vi "Drive Controller.vi"(8 "error in":errorcluster) -> ()   [LabVIEW 2015]
doc: "This VI executes continuously carrying out the current operation and responding to updates or new operation requests. It will often contain the timing or control code that is difficult to place directly in TeleOp. This VI generally opens all sensors and motors and isolates the rest of the robot code from knowing implementation details of how the operations are carried out."
uses:
  JoystickData.ctl
  Drive Setpoints.ctl
  Drive Operations.ctl
  Framework/Robot Global Data.vi
  Global Drive Variables.vi
  RobotDriveGlobal.vi
panel:
  out "Waveform Chart":cluster{"output":dbl, "Angle":dbl, "Yaw":dbl}(graph)
  out "Setpoints":T1(graph)
  out "Current\nCmd":string
  # "Tip: It may be helpful to observe inputs and sensor values.\nYou may also want to display tuning or debugging controls."
  # "Working PID Values:\nP:\nI:\nD:\nF:\nIZ:\nRR:"
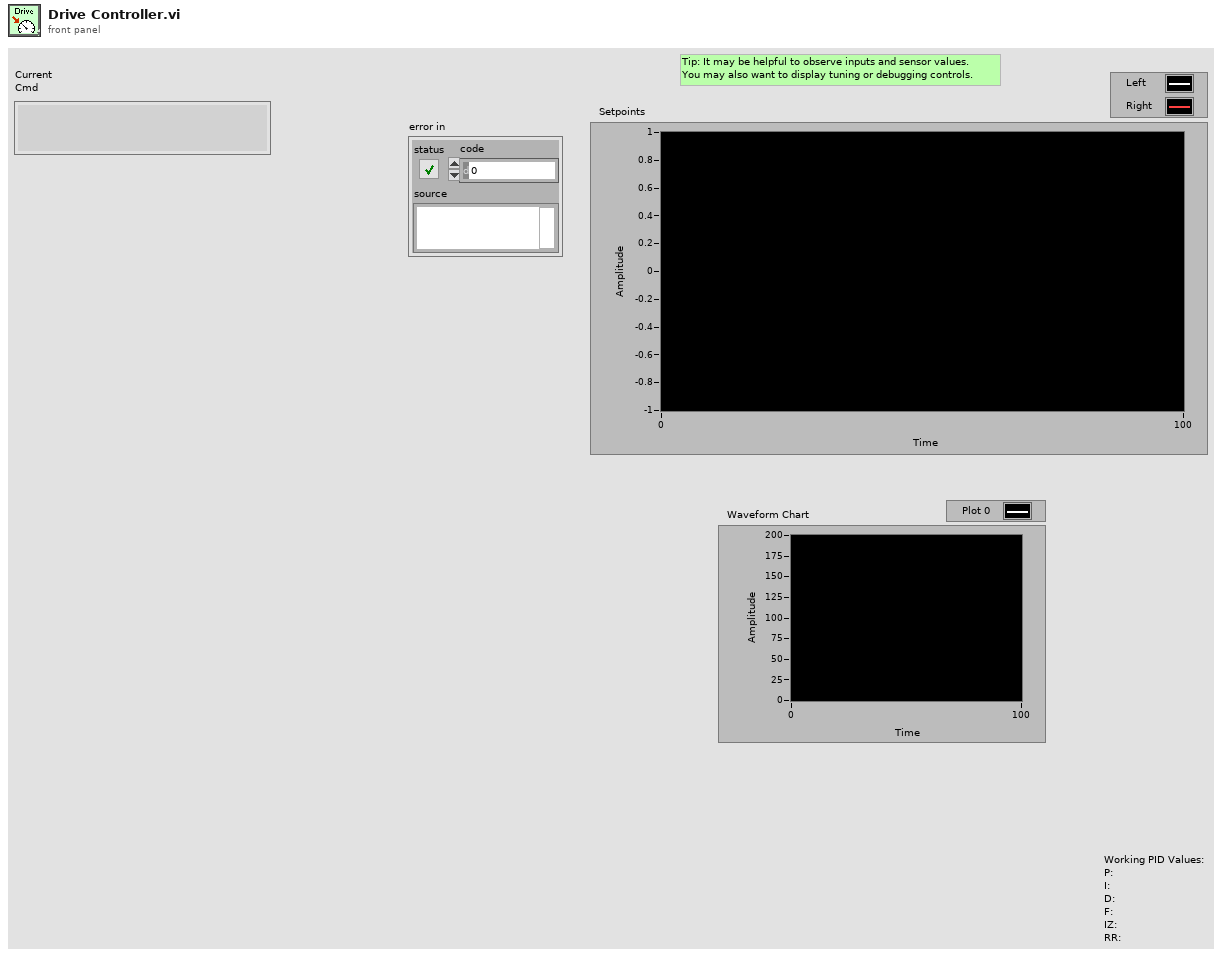
[diagram p1: front panel]
types:
  T1 = cluster{"Left Setpoint":dbl, "Right Setpoint":dbl}
  T2 = typedef "Robot Type Def.ctl" = enum32{"Disabled", "Ghost", "Casper", "Lofty", "Board", "RaceRobot"}
  T3 = typedef "JoystickData.ctl" = cluster{"Axes":dbl[], "Buttons":bool[]}
  T4 = typedef "WPI_JoystickDevRef.ctl" = cluster{"Device":T5}
  T5 = typedef "WPI_JoystickDeviceEnum.ctl" = enum16{"USB 0", "USB 1", "USB 2", "USB 3", "USB 4", "USB 5"}
  T6 = typedef "JoystickMap.ctl" = cluster{"Button ID":dbl, "Joystick ID":dbl}
  T7 = typedef "Drive Setpoints.ctl" = cluster{"Operation":T8, "Left Setpoint":dbl, "Right Setpoint":dbl, "Duration":dbl, "Angle":dbl, "Distance (in)":dbl}
  T8 = typedef "Drive Operations.ctl" = enum16{"Reserve", "Read Current", "Immediate", "Drive for Time", "Drive for Distance", "Turn Degrees"}
  T9 = typedef "Command Status Info.ctl" = cluster{"Name":string, "Status":T10, "notifier out":T11}
  T10 = typedef "Completion Status.ctl" = enum16{"Successful", "Aborted", "Incomplete"}
  T11 = typedef "Completion Notifier.ctl" = refnum<notifier>
  T12 = cluster{"SubSystem Data":T7, cluster{"Start Time (ms)":u32, "Iterations":i32}, cluster{"Command Info":T9, "Description":string, "SubSystem Data":T7, "notifier out":refnum<notifier>, "Subsystem Name":string}}
  T13 = typedef "RobotDrive Type Def.ctl" = cluster{"RobotDriveDevRef":cluster{"DevStatus":errorcluster, "Motors[]":T14[], "Square Inputs":bool, "Max Output":dbl}, "Control Mode":T20, "Motor Settings":T21, "Default Control Mode":T20}
  T14 = typedef "WPI_MotorControlDeviceRef.ctl" = cluster{"DeviceStatus":errorcluster, "Type":T15, "PWM":cluster{"PWM Channel":T16, "DeadBand":T17}, "CAN":cluster{"Device Number":u8, "Control Mode":T18, "Semaphore":T19, "Max Vout":dbl, "TalonSRX Control Mode":T20}, "Invert":bool}
  T15 = typedef "WPI_MotorControlType.ctl" = enum16{"PWM", "CAN", "CANTalonSRX"}
  T16 = typedef "FPGA_DIOPWMChannel.ctl" = enum8{"PWM 0", "PWM 1", "PWM 2", "PWM 3", "PWM 4", "PWM 5", "PWM 6", "PWM 7", "PWM 8", "PWM 9", "PWM MXP 0", "PWM MXP 1", "PWM MXP 2", "PWM MXP 3", "PWM MXP 4", "PWM MXP 5", "PWM MXP 6", "PWM MXP 7", "PWM MXP 8", "PWM MXP 9", "Invalid"}
  T17 = typedef "WPI_PWMDeadband.ctl" = cluster{"Name":string, "maxPositivePwm":i32, "minPositivePwm":i32, "centerPwm":i32, "maxNegativePwm":i32, "minNegativePwm":i32, "angularRange":u16}
  T18 = typedef "WPI_CANJaguar_ControlMode.ctl" = enum8{"Percent VBus", "Current", "Speed", "Position", "Voltage"}
  T19 = typedef "Semaphore RefNum" = refnum<k1>
  T20 = typedef "WPI_CANTalonSRX_APIControlMode.ctl" = enum8{"Percent VBus", "Speed", "Position", "Slave", "Unchanged / Invalid", "Voltage Compensation", "Current", "Motion Profile"}
  T21 = typedef "Drive Motor Settings.ctl" = cluster{"Wheel Radius":dbl, "Encoder Ticks Per Rev":dbl, "Gear Ratio":dbl, "ClimbRev":dbl}
  T22 = typedef "WPI_DriverStationRobotMode2.ctl" = enum16{"Autonomous Disabled", "Autonomous Enabled", "Teleop Disabled", "Teleop Enabled", "Disconnected", "Finish", "Test Disabled", "Test Enabled", "Emergency Stopped"}
  T23 = cluster{"Left Setpoint":dbl, "Left Setpoint":dbl}
  T24 = cluster{"SubSystem Data":T7, cluster{"Start Time (ms)":u32, "Iterations":i32}, "Default Command Arguments":cluster{"Command Info":T9, "Description":string, "SubSystem Data":T7, "notifier out":refnum<notifier>, "Subsystem Name":string}}
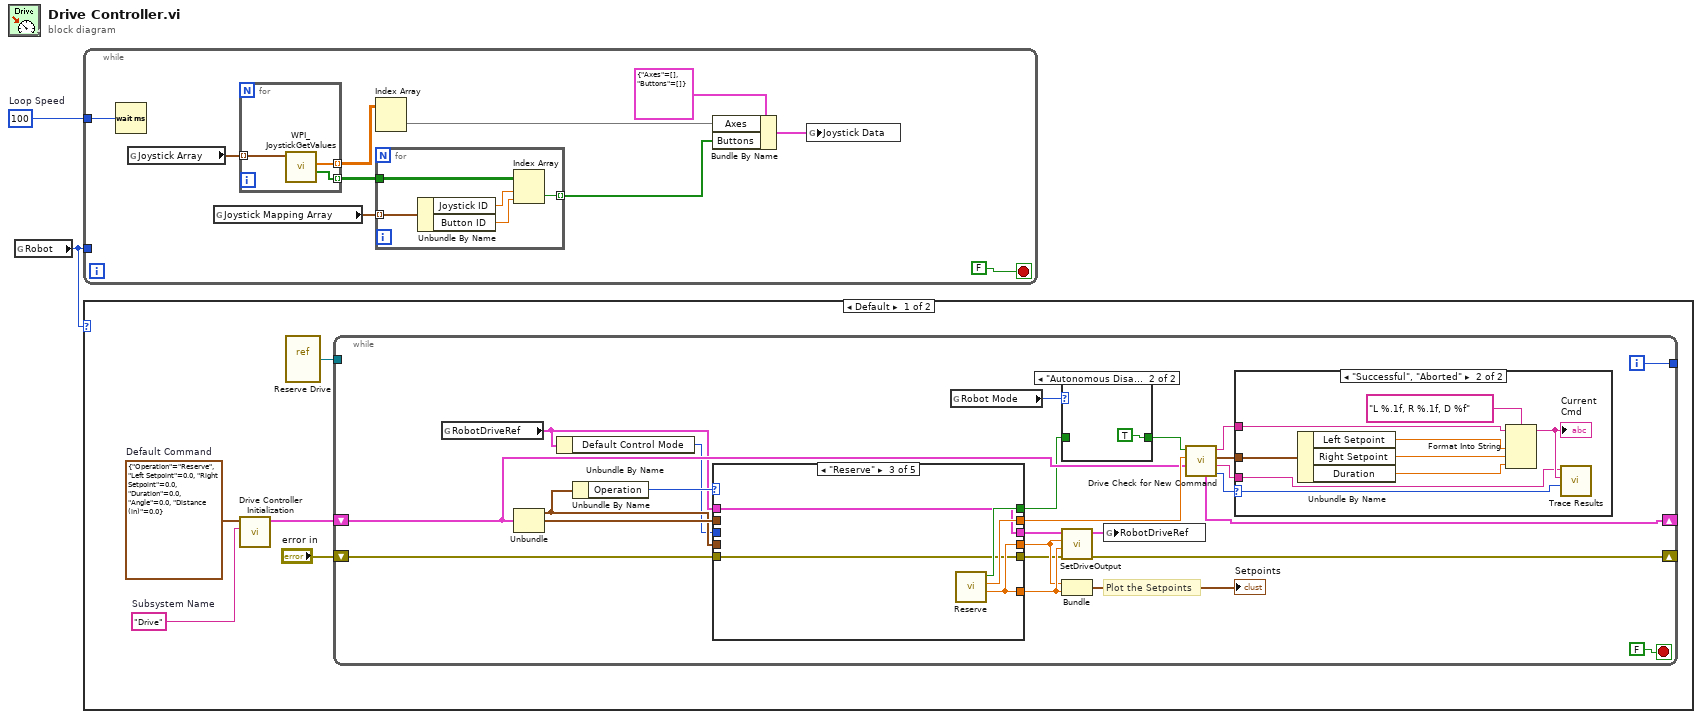
[diagram p0: block diagram]
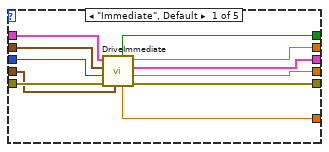
[diagram p4: hidden frame]
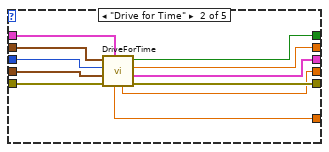
[diagram p5: hidden frame]
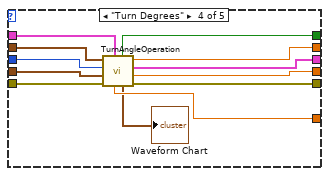
[diagram p6: hidden frame]
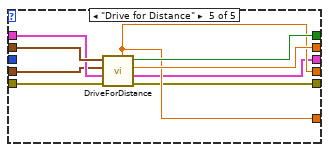
[diagram p7: hidden frame]
diagram:
  w1 = u32 100  # Loop Speed
  n1 = global read "Robot Global Data.vi" "Robot"() -> (w2:T2)
  n2 = while {
    tunnel: w2 -> [_]
    tunnel: w1 -> [w3]
    stop <- FALSE stop-if-true
    n3 = Wait (ms)(milliseconds to wait=w3) -> ()  [unwired: 1 out]
    n4 = global read "Robot Global Data.vi" "Joystick Array"() -> (w8:T4[])
    n5 = global read "Robot Global Data.vi" "Joystick Mapping Array"() -> (w9:T6[])
    n6 = for {
      tunnel: w8 -> [w15] mode=indexing
      tunnel: [w14] -> w7 mode=indexing
      tunnel: [w13] -> w5 mode=indexing
      n7 = call <vilib>:"WPI_JoystickGetValues.vi"("JoystickDevRef"=w15) -> ("Buttons"=w13:bool[], "Axes"=w14:dbl[])  [unwired: 6 in, 3 out]
    }
    n8 = Index Array(array=w7) -> (element=w6:dbl[])  [unwired: 2 in]
    n9 = for {
      tunnel: w9 -> [w20] mode=indexing
      tunnel: w5 -> [w19]
      tunnel: [w16] -> w4 mode=indexing
      n10 = Unbundle By Name(w20) -> ("Joystick ID"=w18:dbl, "Button ID"=w17:dbl)
      n11 = Index Array(array=w19, index (row)=w18, index (col)=w17) -> (element=w16:bool)
    }
    n12 = Bundle By Name(cluster=T3 {"Axes"=[], "Buttons"=[]} ("Joystick Data"), "Axes"=w6, "Buttons"=w4) -> (w10:T3)
    n13 = global write "Global Drive Variables.vi" "Joystick Data"(w10) -> ()
  }
  n14 = case shown="Default" w2 {
    frame Default {
      w24 = T7 {"Operation"=enum."Reserve", "Left Setpoint"=0.0, "Right Setpoint"=0.0, "Duration"=0.0, "Angle"=0.0, "Distance (in)"=0.0}  # Default Command
      w25 = "Drive"  # Subsystem Name
      n15 = call "Drive Controller Initialization.vi"("Subsystem Name"=w25, "Default Command"=w24) -> ("output cluster"=w23:T12)  [unwired: 9 in]
      n16 = vi-ref "Reserve Drive.vi"() -> (w22:refnum<vi>)
      n17 = while {
        shift-right: [w45] -> _
        shift-left: w23 -> [w32]
        tunnel: [w49] -> _
        tunnel: w22 -> [_]
        shift-right: [w34] -> _
        shift-left: "error in" -> [w36]
        i -> [w49]
        stop <- FALSE stop-if-true
        # "Plot the Setpoints"
        n18 = global read "RobotDriveGlobal.vi" "RobotDriveRef"() -> (w27:T13)
        n19 = Unbundle(w32) -> ("SubSystem Data"=w33:T7, w40:cluster{"Start Time (ms)":u32, "Iterations":i32})  [unwired: 1 out]
        n20 = Unbundle By Name(w27) -> ("Default Control Mode"=w26:T20)
        n21 = Unbundle By Name(w33) -> ("Operation"=w47:T8)
        n22 = case shown="\"Reserve\"" w47 {
          tunnel: [w72 w81 w88 w94 w109] -> w44
          tunnel: [w71 w82 w87 w91 w108] -> w30
          tunnel: w40 -> [w70 w83 _ w95 w106]
          tunnel: [w63 w74 w86 w100 w107] -> w38
          tunnel: [w62 w73 w86 w99 w107] -> w39
          tunnel: w27 -> [w69 w80 w85 w98 w105]
          tunnel: w26 -> [w68 w79 _ w97 _]
          tunnel: [w67 w78 w85 w96 w104] -> w37
          tunnel: w36 -> [w66 w77 w84 w93 w103]
          tunnel: [w65 w76 w84 w92 w102] -> w35
          tunnel: w33 -> [w64 w75 _ w90 w101]
          frame "Immediate", Default {
            n23 = call "DriveImmediate.vi"("SubSystem Data"=w64, "error in (no error)"=w66, "Control Mode"=w68, "Cluster"=w70, "RobotDriveRef"=w69) -> ("error out"=w65:errorcluster, "Left Setpoint"=w63:dbl, "RobotDriveRef Out"=w67:T13, "Wait"=w72:dbl, "Right Setpoint"=w62:dbl, "Boolean"=w71:bool)  [unwired: 1 in]
          }
          frame "Drive for Time" {
            n24 = call "DriveForTime.vi"("RobotDriveRef"=w80, "error in (no error)"=w77, "SubSystem Data"=w75, "Control Mode"=w79, "Cluster"=w83) -> ("error out"=w76:errorcluster, "RobotDriveRef Out"=w78:T13, "Wait"=w81:dbl, "Finished"=w82:bool, "Left Setpoint"=w74:dbl, "Right Setpoint"=w73:dbl)  [unwired: 1 in]
          }
          frame "Reserve" {
            n25 = call "Reserve.vi"() -> ("Don't move motors while reserved"=w86:dbl, "Numeric"=w88:dbl, "ignore previous (F)"=w87:bool)  [unwired: 9 in]
          }
          frame "Turn Degrees" {
            n26 = call "TurnAngleOperation.vi"("RobotDriveRef in"=w98, "error in (no error)"=w93, "SubSystem Data"=w90, "Control Mode"=w97, "Command Loop Data"=w95) -> ("error out"=w92:errorcluster, "Left Motor Value"=w100:dbl, "RobotDriveRef out"=w96:T13, "Wait Time"=w94:dbl, "Waveform Chart"=→"Waveform Chart":cluster{"output":dbl, "Angle":dbl, "Yaw":dbl}, "Finished"=w91:bool, "Right Motor Value"=w99:dbl)
          }
          frame "Drive for Distance" {
            n27 = call "DriveForDistance.vi"("error in (no error)"=w103, "RobotDriveRef"=w105, "SubSystem Data"=w101, "Command Loop Data"=w106) -> ("error out"=w102:errorcluster, "RobotDriveRef Out"=w104:T13, "Wait Time"=w109:dbl, "Finished"=w108:bool, "Left Setpoint"=w107:dbl)  [unwired: 3 in]
          }
        }
        n28 = global read "Robot Global Data.vi" "Robot Mode"() -> (w31:T22)
        n29 = case shown="\"Autonomous Disabled\", \"Teleop Disabled\"" w31 {
          tunnel: w30 -> [w51 _]
          tunnel: [w51 TRUE] -> w29
          frame Default {
          }
          frame "Autonomous Disabled", "Teleop Disabled" {
          }
        }
        n30 = call "SetDriveOutput.vi"("error in (no error)"=w35, "RightSpeed"=w39, "LeftSpeed"=w38, "RobotDriveRef In"=w37) -> ("error out"=w34:errorcluster, "RobotDriveRef Out"=w28:T13)  [unwired: 5 in, 1 out]
        n31 = Bundle("Left Setpoint"=w38, "Left Setpoint"=w39) -> (→"Setpoints":T23)  [unwired: 1 in]
        n32 = global write "RobotDriveGlobal.vi" "RobotDriveRef"(w28) -> ()
        n33 = call "Drive Check for New Command.vi"("input cluster"=w32, "Wait time (ms)"=w44, "Finished?"=w29) -> ("Completion"=w46:T10, "Subsystem Name"=w41:string, "SetPoint"=w42:T7, "Initial Trace String"=w43:string, "output cluster"=w45:T24)  [unwired: 4 in]
        n34 = case shown="\"Successful\", \"Aborted\"" w46 {
          selector: w46 -> [_ w61]
          tunnel: w43 -> [_ w56]
          tunnel: w42 -> [_ w57]
          tunnel: w41 -> [_ w53]
          frame "Incomplete", Default {
            # "Continuing current command"
          }
          frame "Successful", "Aborted" {
            # "Report and setup for next command"
            n35 = Unbundle By Name(w57) -> ("Left Setpoint"=w59:dbl, "Right Setpoint"=w60:dbl, "Duration"=w54:dbl)
            n36 = Format Into String(format string="L %.1f, R %.1f, D %f", initial string=w56, w59, w60, w54) -> (resulting string=w55:string)  [unwired: 1 in, 1 out]
            "Current\nCmd" <- w55
            n37 = call <vilib>:"Trace Results.vi"("Status of previous command"=w61, "Description"=w55, "Subsystem"=w53) -> ()  [unwired: 9 in]
          }
        }
      }
    }
    frame "Board" {
    }
  }
